vi "escaping test.vi"() -> ()   [LabVIEW 2014]
uses:
  generate string.vi
  json generator.lvlib
panel:
  out "xml string":string
  out "element":i32
  out "mine":string
  out "json":string
  out "data":cluster{u8, u8}[](array[cluster]) {"?" format="%.0b"; "?" format="%.0b"}
  out "mine":string
  out "json string":string
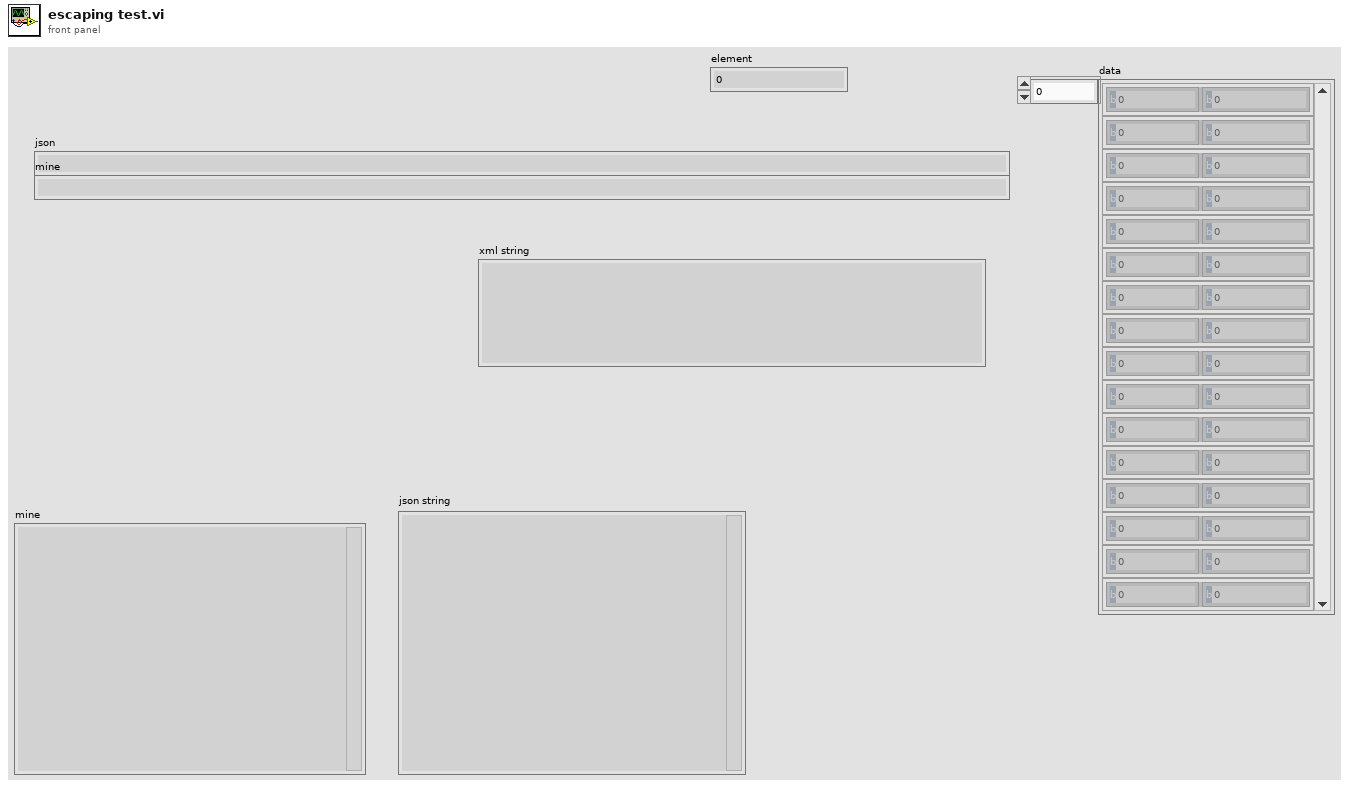
[diagram p1: front panel]
types:
  T1 = cluster{bool, i32, string, "result string":string}
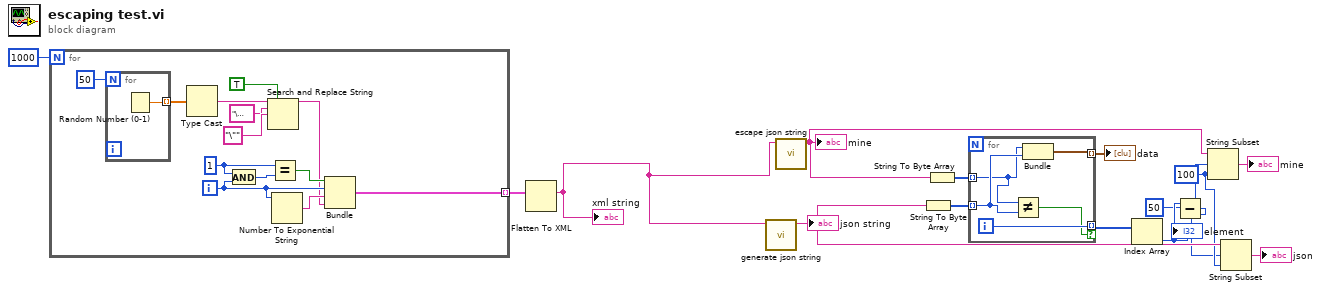
[diagram p0: block diagram]
diagram:
  w4 = 100 ("length (rest)")
  n1 = for {
    N: 1000 -> [_]
    tunnel: [w23] -> w14 mode=indexing
    i -> [w27]
    w25 = 1 ("x")
    n2 = for {
      N: 50 -> [_]
      tunnel: [w29] -> w22 mode=indexing
      n3 = Random Number (0-1)() -> (number: 0 to 1=w29:dbl)
    }
    n4 = Type Cast(x=w22) -> (*(type *) &x=w20:string)  [unwired: 1 in]
    n5 = And(x=w25, y=w27) -> (x .and. y?=w26:i32)
    n6 = Search and Replace String(replace all?=TRUE ("replace all? (F)"), input string=w20, search string="\u0000", replace string="\"" ("replace string (\"\")")) -> (result string=w19:string)  [unwired: 4 in, 3 out]
    n7 = Equal?(x=w25, y=w26) -> (x = y?=w24:bool)
    n8 = Number To Exponential String(number=w27) -> (E-format string=w28:string)  [unwired: 3 in]
    n9 = Bundle(w24, w27, w28, "result string"=w19) -> (w23:T1)  [unwired: 1 in]
  }
  n10 = Flatten To XML(anything=w14) -> (xml string=w13:string)
  "xml string" <- w13
  n11 = call-poly "generate json string.vi"("base string"=w13) -> ("json string"=w7:string)  [unwired: 10 in]
  "json string" <- w7
  n12 = call "escape json string.vi"("base string"=w13) -> ("String out"=w8:string)  [unwired: 10 in]
  "mine" <- w8
  n13 = String To Byte Array(string=w7) -> (unsigned byte array=w12:u8[])
  n14 = String To Byte Array(string=w8) -> (unsigned byte array=w11:u8[])
  n15 = for {
    tunnel: w12 -> [w34] mode=indexing
    tunnel: w11 -> [w33] mode=indexing
    tunnel: [w32] -> w10 mode=indexing
    tunnel: [w31] -> w9 mode=indexing if=w30
    i -> [w31]
    n16 = Not Equal?(x=w33, y=w34) -> (x != y?=w30:bool)
    n17 = Bundle(w33, w34) -> (w32:cluster{u8, u8})  [unwired: 1 in]
  }
  "data" <- w10
  n18 = Index Array(array=w9) -> (element=w6:i32)  [unwired: 1 in]
  "element" <- w6
  n19 = Subtract(x=w6, y=50) -> (x-y=w3:i32)
  n20 = String Subset(string=w8, offset (0)=w3, length (rest)=w4) -> (substring=→"mine":string)
  n21 = String Subset(string=w7, offset (0)=w3, length (rest)=w4) -> (substring=→"json":string)
